vi "ImportExcelValues.vi"(8 "error in (no error)":errorcluster, 10 "excel_path":path, 11 "Excel in":refnum<class "Excel.lvclass">) -> (0 "error out":errorcluster, 3 "Excel out":refnum<class "Excel.lvclass">)   [LabVIEW 2015, in "Excel.lvclass"]
uses:
  Excel.lvclass
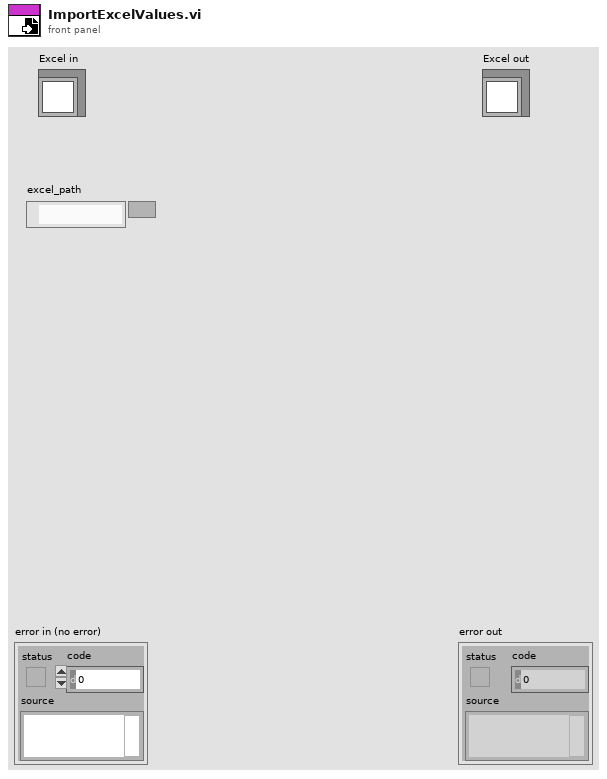
[diagram p1: front panel]
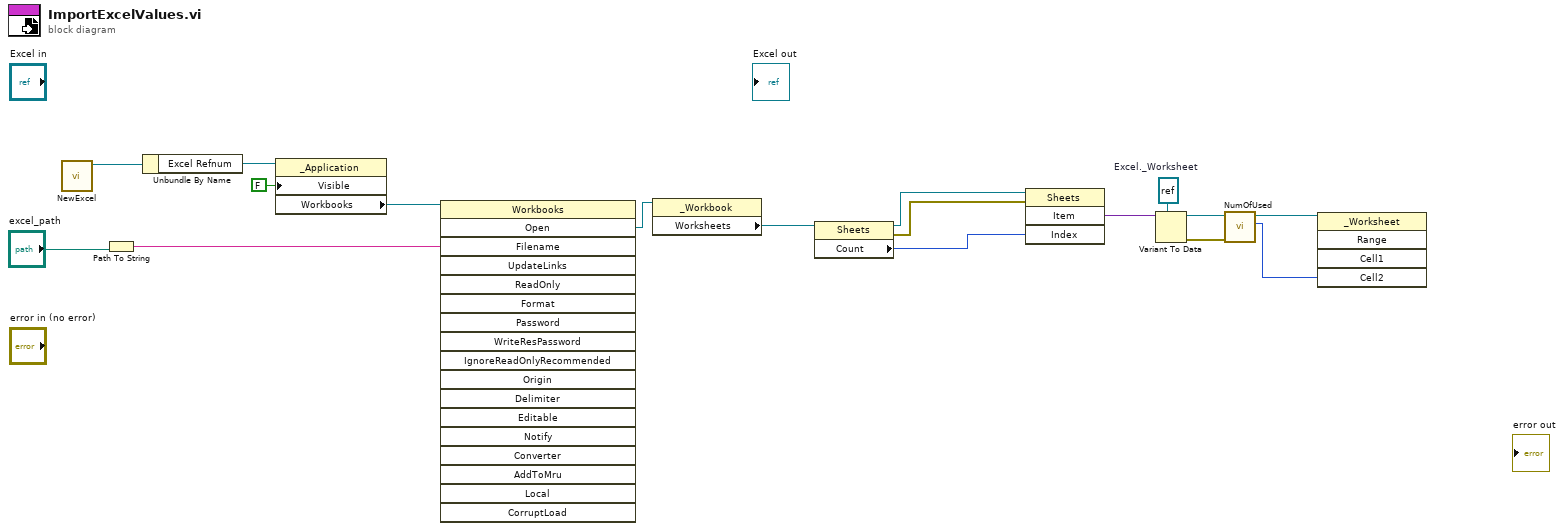
[diagram p0: block diagram]
diagram:
  w7 = refnum<k7> refnum  # Excel._Worksheet
  n1 = call "NewExcel.vi"() -> ("Excel out"=w17:refnum<class "Excel.lvclass">)  [unwired: 10 in, 1 out]
  n2 = Path To String(path="excel_path") -> (string=w12:string)
  n3 = Unbundle By Name(w17) -> ("Excel Refnum"=w16:refnum<k7>)
  n4 = property class="_Application"(reference=w16, "Visible"=FALSE) -> ("Workbooks"=w14:refnum<k7>)  [unwired: 1 in, 2 out]
  n5 = invoke class="Workbooks" method="Open"(reference=w14, "Filename"=w12) -> ("Open"=w11:refnum<k7>)  [unwired: 16 in, 17 out]
  n6 = property class="_Workbook"(reference=w11) -> ("Worksheets"=w10:refnum<k7>)  [unwired: 1 in, 2 out]
  n7 = property class="Sheets"(reference=w10) -> (reference out=w9:refnum<k7>, error out=w8:errorcluster, "Count"=w3:i32)  [unwired: 1 in]
  n8 = invoke class="Sheets" method="Item"(reference=w9, error in=w8, "Index"=w3) -> ("Item"=w6:variant)  [unwired: 1 in, 3 out]
  n9 = Variant To Data(type=w7, Variant=w6) -> (data=w5:refnum<k7>, error out=w4:errorcluster)  [unwired: 1 in]
  n10 = call "NumOfUsed.vi"("error in (no error)"=w4, "worksheet_Refnum"=w5) -> ("Columns(0)"=w1:i32, "worksheet_Refnum"=w2:refnum<k7>)  [unwired: 6 in, 2 out]
  n11 = invoke class="_Worksheet" method="Range"(reference=w2, "Cell2"=w1) -> ()  [unwired: 3 in, 5 out]
